vi "Set and Print Serial Wire Mode to Console.vi"(8 "error in (no error)":errorcluster, 10 "Wire Mode":i16, 11 "VISA Refnum in":refnum<visa-resource-name>) -> (0 "error out":errorcluster, 3 "VISA Refnum out":refnum<visa-resource-name>)   [LabVIEW 2021, in "Modbus Master Engine.lvlib"]
uses:
  Modbus Master Engine.lvlib
  <vilib>/NI VeriStand/Custom Device Tools/Custom Device Utility Library/Custom Device Utility Library.lvlib
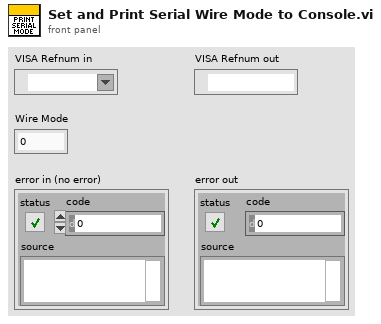
[diagram p1: front panel]
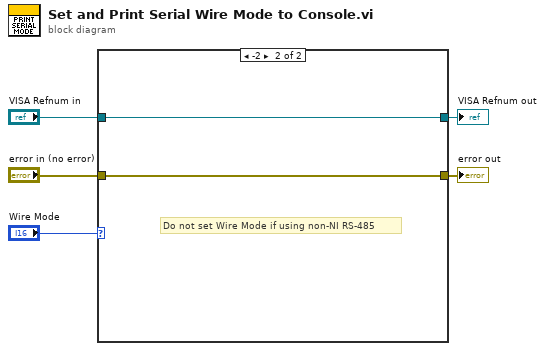
[diagram p0: block diagram]
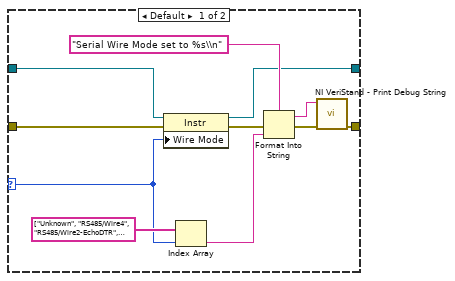
[diagram p2: hidden frame]
diagram:
  n1 = case shown="-2" "Wire Mode" {
    selector: "Wire Mode" -> [w6 _]
    tunnel: [w12 w17] -> w5
    tunnel: "VISA Refnum in" -> [w9 w18]
    tunnel: [w8 w18] -> w3
    tunnel: "error in (no error)" -> [w7 w17]
    frame Default {
      n2 = property class="Instr"(reference=w9, error in=w7, "Wire Mode"=w6) -> (reference out=w8:refnum<visa-resource-name>, error out=w13:errorcluster)
      n3 = Index Array(array=string[] ["Unknown", "RS485/Wire4", "RS485/Wire2-EchoDTR", "RS485/Wire2-CtrlDTR", "RS485/Wire2-Auto", "RS232/DTE", "RS232/DCE", "RS232/AUTO"] ("Strings []"), index=w6) -> (element=w16:string)
      n4 = Format Into String(format string="Serial Wire Mode set to %s\\n", error in=w13, w16) -> (resulting string=w11:string, error out=w14:errorcluster)  [unwired: 1 in]
      n5 = call <vilib>:"NI VeriStand - Print Debug String.vi"("error in (no error)"=w14, "Message"=w11) -> ("error out"=w12:errorcluster)  [unwired: 9 in]
    }
    frame -2 {
      # "Do not set Wire Mode if using non-NI RS-485"
    }
  }
  "error out" <- w5
  "VISA Refnum out" <- w3
